vi "Write Paths.vi"(8 "error in (no error)":errorcluster, 10 "Paths":refnum<class "Path.lvclass">[](array[class]), 11 "Cable Path Group in":refnum<class "Path Group.lvclass">) -> (0 "error out":errorcluster, 3 "Cable Path Group out":refnum<class "Path Group.lvclass">)   [LabVIEW 2023, in "RFCalAndFixtureCharact.Common.lvlib" / "Path Group.lvclass"]
uses:
  Path Group.lvclass
  Path/Path.lvclass
  Path Group.lvclass/Path Group.ctl
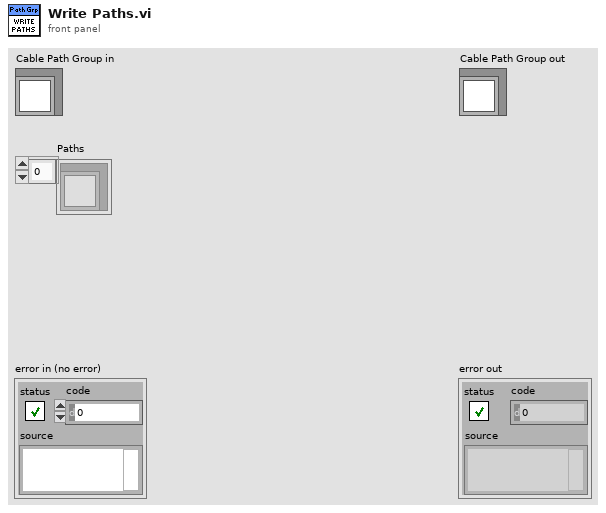
[diagram p1: front panel]
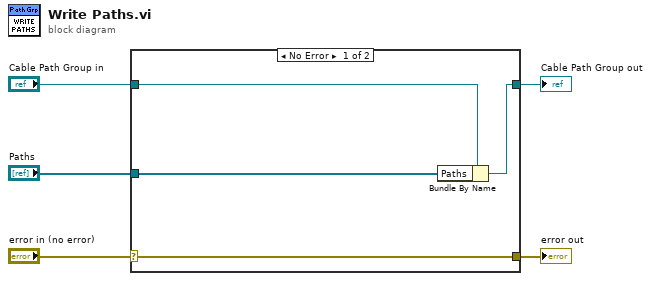
[diagram p0: block diagram]
diagram:
  n1 = case shown="No Error" "error in (no error)" {
    selector: "error in (no error)" -> [w9 w10]
    tunnel: [w9 w10] -> w4
    tunnel: [w7 w11] -> w2
    tunnel: "Cable Path Group in" -> [w8 w11]
    tunnel: "Paths" -> [w6 _]
    frame No Error {
      n2 = Bundle By Name(cluster=w8, "Paths"=w6) -> (w7:refnum<class "Path Group.lvclass">)
    }
    frame Error {
    }
  }
  "error out" <- w4
  "Cable Path Group out" <- w2
